vi "Application User Name.vi"(8 "Error In":errorcluster) -> (0 "Error Out":errorcluster, 3 "User Name":string)   [LabVIEW 2017, in "Eulogy.lvlib"]
uses:
  Eulogy.lvlib
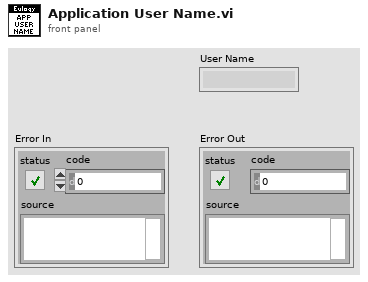
[diagram p1: front panel]
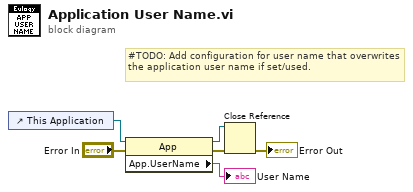
[diagram p0: block diagram]
diagram:
  # "#TODO: Add configuration for user name that overwrites the application user name if set/used."
  n1 = control-ref of="This Application"() -> (w1:refnum<vi>)
  n2 = property class="App"(reference=w1, error in="Error In") -> (reference out=w6:refnum<vi>, error out=w3:errorcluster, "App.UserName"=→"User Name":string)
  n3 = Close Reference(reference=w6, error in (no error)=w3) -> (error out=→"Error Out":errorcluster)
